vi "Command.vi"(8 "error in (no error)":errorcluster, 9 "command data":u8[](array[numeric]), 10 "node":u8, 11 "ProPar in":refnum<class "PL Bronkhorst ProPar.lvclass">) -> (0 "error out":errorcluster, 2 "response data":u8[](array[numeric]), 3 "ProPar out":refnum<class "PL Bronkhorst ProPar.lvclass">)   [LabVIEW 2015, in "PL Bronkhorst ProPar.lvclass"]
doc: "Sends specified <b>command data</b> to specified <b>node</b> and returns <b>response data</b>."
uses:
  PL Bronkhorst ProPar.lvclass
  PL Bronkhorst ProPar.lvclass/PL Bronkhorst ProPar.ctl
panel:
  out "response":u8[](array[numeric])
  out "header":u8[](array[numeric])
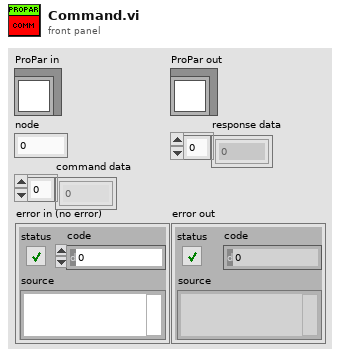
[diagram p1: front panel]
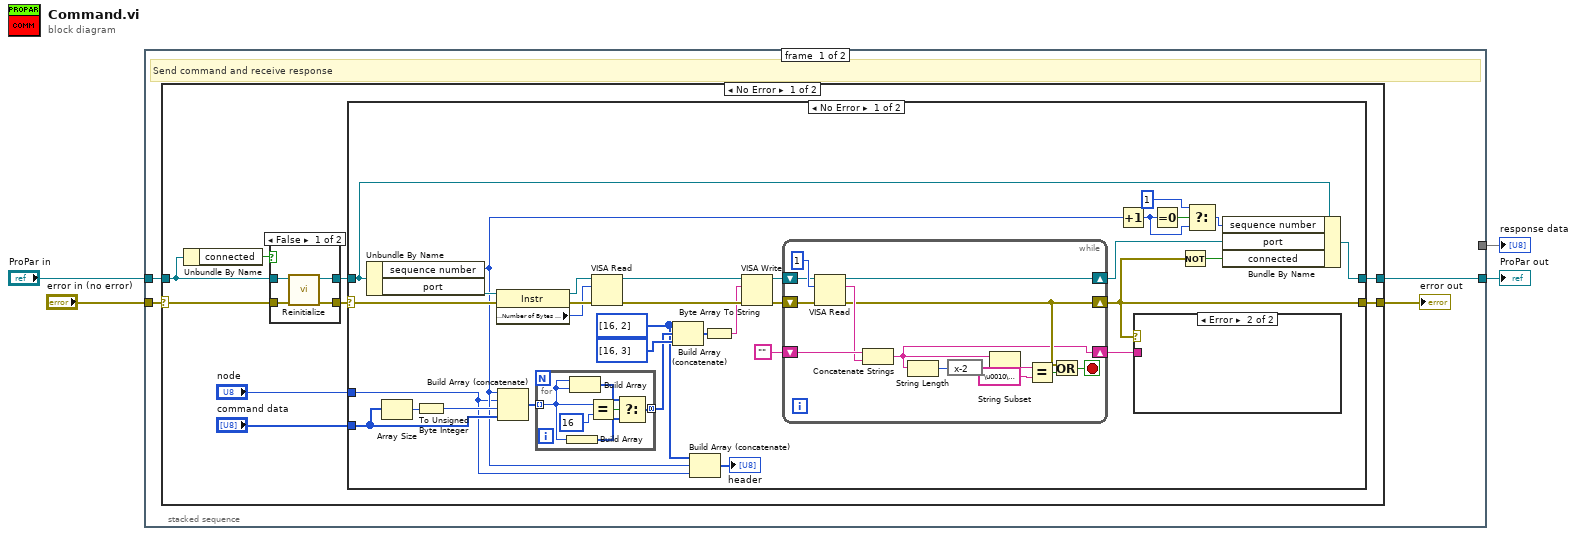
[diagram p0: block diagram]
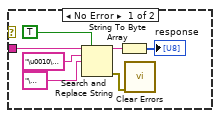
[diagram p2: hidden frame]
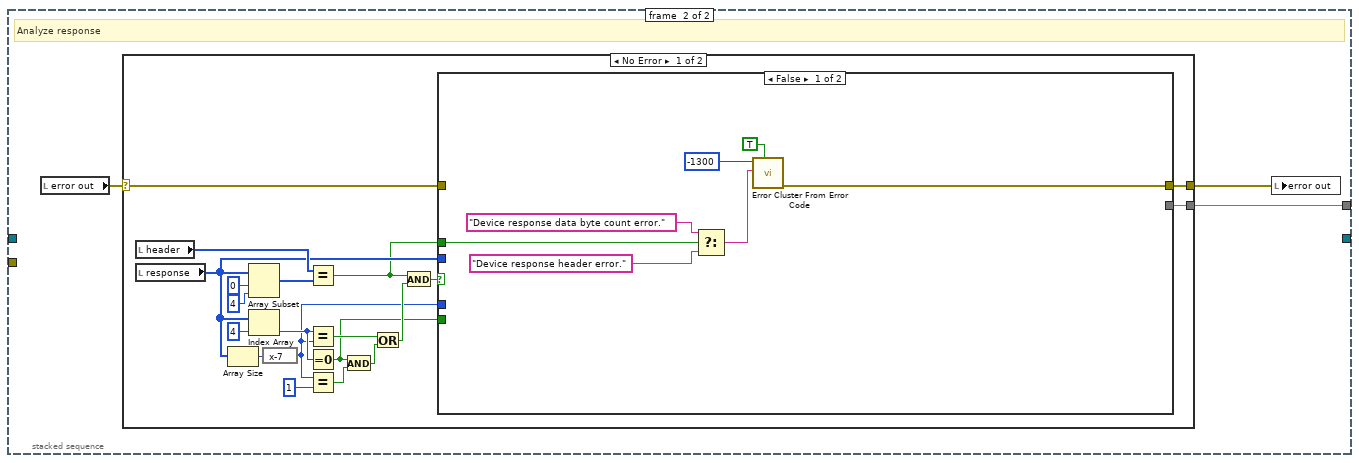
[diagram p6: hidden frame]
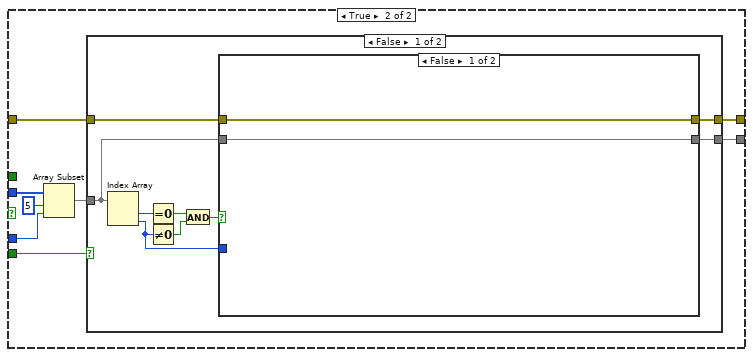
[diagram p7: hidden frame]
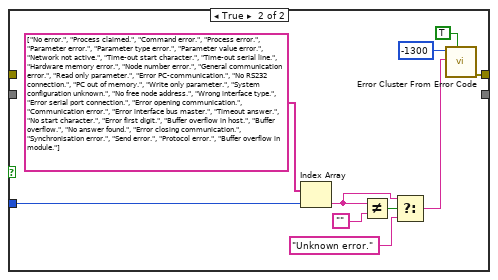
[diagram p8: hidden frame]
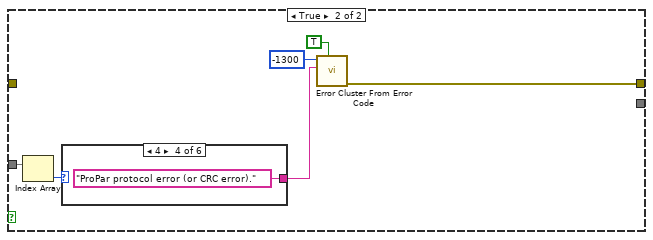
[diagram p9: hidden frame]
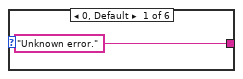
[diagram p10: hidden frame]
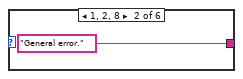
[diagram p11: hidden frame]
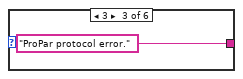
[diagram p12: hidden frame]
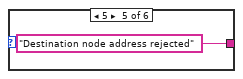
[diagram p13: hidden frame]
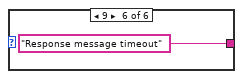
[diagram p14: hidden frame]
diagram:
  n1 = stacked-sequence {
    tunnel: "ProPar in" -> [w8 _]
    tunnel: "error in (no error)" -> [w7 _]
    tunnel: [w6 _] -> w2
    tunnel: [_ w87] -> w1
    frame #0 {
      # "Send command and receive response"
      n2 = case shown="No Error" w7 {
        selector: w7 -> [w15 w86]
        tunnel: w8 -> [w16 w85]
        tunnel: [w12 w86] -> w5
        tunnel: [w11 w85] -> w6
        frame No Error {
          n3 = Unbundle By Name(w16) -> ("connected"=w17:bool)
          n4 = case shown="False" w17 {
            tunnel: w16 -> [w82 w84]
            tunnel: w15 -> [w81 w83]
            tunnel: [w80 w84] -> w13
            tunnel: [w79 w83] -> w14
            frame False {
              n5 = call "Reinitialize.vi"("error in (no error)"=w81, "ProPar in"=w82) -> ("error out"=w79:errorcluster, "ProPar out"=w80:refnum<class "PL Bronkhorst ProPar.lvclass">)  [unwired: 8 in]
            }
            frame True {
            }
          }
          n6 = case shown="No Error" w14 {
            selector: w14 -> [w41 w78]
            tunnel: w13 -> [w49 w77]
            tunnel: [w20 w78] -> w12
            tunnel: [w48 w77] -> w11
            tunnel: "node" -> [w18 _]
            tunnel: "command data" -> [w24 _]
            frame No Error {
              w23 = u8[] [16, 2]
              n7 = Unbundle By Name(w49) -> ("sequence number"=w19:u8, "port"=w42:refnum<visa-resource-name>)
              n8 = Array Size(array=w24) -> (size(s)=w47:i32)
              n9 = To Unsigned Byte Integer(number=w47) -> (unsigned 8bit integer=w25:u8)
              n10 = property class="Instr"(reference=w42, error in=w41) -> (reference out=w40:refnum<visa-resource-name>, error out=w39:errorcluster, "Serial Settings:Number of Bytes at Serial Port"=w38:u32)
              n11 = Build Array (concatenate)(w19, w18, w25, w24) -> (w26:u8[])
              n12 = for {
                tunnel: w26 -> [w73] mode=indexing
                tunnel: [w71] -> w27 mode=concatenating
                n13 = Build Array(w73) -> (w74:u8[])
                n14 = Build Array(w73, w73) -> (w72:u8[])
                n15 = Equal?(x=w73, y=u8 16) -> (x = y?=w75:bool)
                n16 = Select(t=w72, s=w75, f=w74) -> (s? t:f=w71:u8[])
              }
              n17 = VISA Read(VISA resource name=w40, byte count=w38, error in (no error)=w39) -> (VISA resource name out=w37:refnum<visa-resource-name>, error out=w36:errorcluster)  [unwired: 2 out]
              n18 = Build Array (concatenate)(w23, w27, u8[] [16, 3]) -> (w35:u8[])
              n19 = Build Array (concatenate)(w23, w19, w18) -> (→"header":u8[])
              n20 = Byte Array To String(unsigned byte array=w35) -> (string=w34:string)
              n21 = VISA Write(VISA resource name=w37, write buffer=w34, error in (no error)=w36) -> (VISA resource name out=w33:refnum<visa-resource-name>, error out=w32:errorcluster)  [unwired: 1 out]
              n22 = while {
                shift-right: [w58] -> w20
                shift-left: w32 -> [w70]
                shift-right: [w69] -> w31
                shift-left: w33 -> [w66]
                shift-right: [w57] -> w21
                shift-left: "" -> [w65]
                stop <- w67 stop-if-true
                n23 = VISA Read(VISA resource name=w66, byte count=u32 1, error in (no error)=w70) -> (VISA resource name out=w69:refnum<visa-resource-name>, read buffer=w64:string, error out=w58:errorcluster)  [unwired: 1 out]
                n24 = Concatenate Strings(w65, w64) -> (w57:string)
                n25 = String Length(string=w57) -> (length=w63:i32)
                n26 = expression code="x-2"(w63) -> (w62:i32)
                n27 = String Subset(string=w57, offset (0)=w62) -> (substring=w61:string)  [unwired: 1 in]
                n28 = Equal?(x=w61, y="\u0010\u0003" ("string")) -> (x = y?=w59:bool)
                n29 = Or(x=w58, y=w59) -> (x .or. y?=w67:bool)
              }
              n30 = Increment(x=w19) -> (x+1=w45:u8)
              n31 = case shown="Error" w20 {
                tunnel: w21 -> [w51 _]
                frame No Error {
                  n32 = Search and Replace String(replace all?=TRUE ("replace all? (F)"), input string=w51, search string="\u0010\u0010" ("string"), replace string="\u0010" ("string")) -> (result string=w53:string, error out=w50:errorcluster)  [unwired: 4 in, 2 out]
                  n33 = String To Byte Array(string=w53) -> (unsigned byte array=→"response":u8[])
                  n34 = call <vilib>:"Clear Errors.vi"("error in (no error)"=w50) -> ()  [unwired: 5 in, 2 out]
                }
                frame Error {
                }
              }
              n35 = Equal To 0?(x=w45) -> (x = 0?=w46:bool)
              n36 = Not(x=w20) -> (.not. x?=w30:bool)
              n37 = Select(t=u8 1, s=w46, f=w45) -> (s? t:f=w43:u8)
              n38 = Bundle By Name(cluster=w49, "sequence number"=w43, "port"=w31, "connected"=w30) -> (w48:refnum<class "PL Bronkhorst ProPar.lvclass">)
            }
            frame Error {
            }
          }
        }
        frame Error {
        }
      }
      "error out" <- w5
    }
    frame #1 {
      # "Analyze response"
      n39 = local read "error out"() -> (w89:errorcluster)
      n40 = case shown="No Error" w89 {
        selector: w89 -> [w94 w158]
        tunnel: [w98 w158] -> w88
        tunnel: [w91 _] -> w87
        frame No Error {
          n41 = local read "header"() -> (w100:u8[])
          n42 = local read "response"() -> (w93:u8[])
          n43 = Array Size(array=w93) -> (size(s)=w104:i32)
          n44 = Array Subset(array=w93, index=0, length=4) -> (w97:u8[])
          n45 = Index Array(array=w93, index=4) -> (element=w95:u8)
          n46 = expression code="x-7"(w104) -> (w92:i32)
          n47 = Equal?(x=w100, y=w97) -> (x = y?=w90:bool)
          n48 = Equal?(x=w95, y=w92) -> (x = y?=w106:bool)
          n49 = Equal To 0?(x=w95) -> (x = 0?=w96:bool)
          n50 = Equal?(x=w92, y=1) -> (x = y?=w108:bool)
          n51 = And(x=w96, y=w108) -> (x .and. y?=w109:bool)
          n52 = Or(x=w106, y=w109) -> (x .or. y?=w105:bool)
          n53 = And(x=w90, y=w105) -> (x .and. y?=w99:bool)
          n54 = case shown="False" w99 {
            tunnel: [w114 w123] -> w98
            tunnel: w93 -> [_ w122]
            tunnel: w96 -> [_ w124]
            tunnel: w92 -> [_ w120]
            tunnel: w94 -> [_ w118]
            tunnel: [_ w117] -> w91
            tunnel: w90 -> [w112 _]
            frame False {
              n55 = Select(t="Device response data byte count error." ("format string"), s=w112, f="Device response header error." ("format string")) -> (s? t:f=w110:string)
              n56 = call <vilib>:"Error Cluster From Error Code.vi"("show call chain? (False)"=TRUE, "error message (\"\")"=w110, "error code (0)"=-1300) -> ("error out"=w114:errorcluster)  [unwired: 6 in]
            }
            frame True {
              n57 = Array Subset(array=w122, index=5, length=w120) -> (w119:u8[])
              n58 = case shown="False" w124 {
                tunnel: [w128 w148] -> w123
                tunnel: w119 -> [w126 w147]
                tunnel: w118 -> [w127 _]
                tunnel: [w125 _] -> w117
                frame False {
                  n59 = Index Array(array=w126) -> (element #1=w133:u8, element #2=w129:u8)  [unwired: 2 in]
                  n60 = Equal To 0?(x=w133) -> (x = 0?=w132:bool)
                  n61 = Not Equal To 0?(x=w129) -> (x != 0?=w131:bool)
                  n62 = And(x=w132, y=w131) -> (x .and. y?=w130:bool)
                  n63 = case shown="False" w130 {
                    tunnel: w129 -> [_ w141]
                    tunnel: [w135 w143] -> w128
                    tunnel: w127 -> [w135 _]
                    tunnel: w126 -> [w134 _]
                    tunnel: [w134 _] -> w125
                    frame False {
                    }
                    frame True {
                      n64 = Index Array(array=string[] ["No error.", "Process claimed.", "Command error.", "Process error.", "Parameter error.", "Parameter type error.", "Parameter value error.", "Network not active.", "Time-out start character.", "Time-out serial line.", "Hardware memory error.", "Node number error.", "General communication error.", "Read only parameter.", "Error PC-communication.", "No RS232 connection.", "PC out of memory.", "Write only parameter.", "System configuration unknown.", "No free node address.", "Wrong interface type.", "Error serial port connection.", "Error opening communication.", "Communication error.", "Error interface bus master.", "Timeout answer.", "No start character.", "Error first digit.", "Buffer overflow in host.", "Buffer overflow.", "No answer found.", "Error closing communication.", "Synchronisation error.", "Send error.", "Protocol error.", "Buffer overflow in module."], index=w141) -> (element=w138:string)
                      n65 = Not Equal?(x=w138, y="") -> (x != y?=w139:bool)
                      n66 = Select(t=w138, s=w139, f="Unknown error.") -> (s? t:f=w136:string)
                      n67 = call <vilib>:"Error Cluster From Error Code.vi"("show call chain? (False)"=TRUE, "error message (\"\")"=w136, "error code (0)"=-1300) -> ("error out"=w143:errorcluster)  [unwired: 6 in]
                    }
                  }
                }
                frame True {
                  n68 = Index Array(array=w147) -> (element=w146:u8)  [unwired: 1 in]
                  n69 = case shown="4" w146 {
                    tunnel: ["Unknown error." ("format string") "General error." ("format string") "ProPar protocol error." ("format string") "ProPar protocol error (or CRC error)." ("format string") "Destination node address rejected" ("format string") "Response message timeout" ("format string")] -> w149
                    frame 0, Default {
                    }
                    frame 1, 2, 8 {
                    }
                    frame 3 {
                    }
                    frame 4 {
                    }
                    frame 5 {
                    }
                    frame 9 {
                    }
                  }
                  n70 = call <vilib>:"Error Cluster From Error Code.vi"("show call chain? (False)"=TRUE, "error message (\"\")"=w149, "error code (0)"=-1300) -> ("error out"=w148:errorcluster)  [unwired: 6 in]
                }
              }
            }
          }
        }
        frame Error {
        }
      }
      n71 = local write "error out"(w88) -> ()
    }
  }
  "ProPar out" <- w2
  "response data" <- w1
